vi "Flush.vi"(11 "TypedCircularBuffer in":refnum<class "LogCircularBuffer.lvclass">) -> (2 "Flushed Buffer":T1[](array[typedef]), 3 "TypedCircularBuffer out":refnum<class "LogCircularBuffer.lvclass">)   [LabVIEW 2024, in "LogCircularBuffer.lvclass"]
uses:
  LogCircularBuffer.lvclass
  Type.ctl
  RQMHCore/ErrorReporting/Record/LogRecord.lvclass
  LogCircularBuffer.lvclass/LogCircularBuffer.ctl
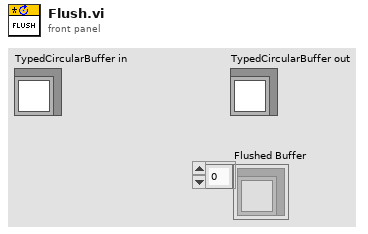
[diagram p1: front panel]
types:
  T1 = typedef "LogCircularBuffer.lvclass/Type.ctl" = refnum<class "LogRecord.lvclass">
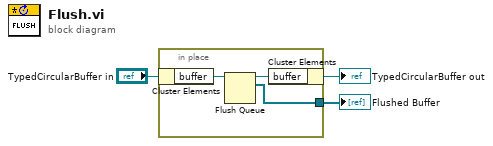
[diagram p0: block diagram]
diagram:
  n1 = in-place {
    in-place-border: [w4] -> w1
    n2 = in-place-cluster #1("TypedCircularBuffer in") -> ("buffer"=w6:refnum<queue>)
    n3 = Flush Queue(queue=w6) -> (queue out=w5:refnum<queue>, remaining elements=w4:T1[])  [unwired: 1 in, 1 out]
    n4 = in-place-cluster #1("buffer"=w5) -> (→"TypedCircularBuffer out":refnum<class "LogCircularBuffer.lvclass">)
  }
  "Flushed Buffer" <- w1
